vi "获取用户UID.vi"(8 "error in (no error)":errorcluster caption="错误输入（无错误）") -> (0 "error out":errorcluster caption="错误输出", 3 "uid":string[](array[string]))   [LabVIEW 2016, in "wxpusher.lvlib"]
uses:
  wxpusher.lvlib
  <vilib>/httpClient/LabVIEWHTTPClient.lvlib
panel:
  out "数据":T1
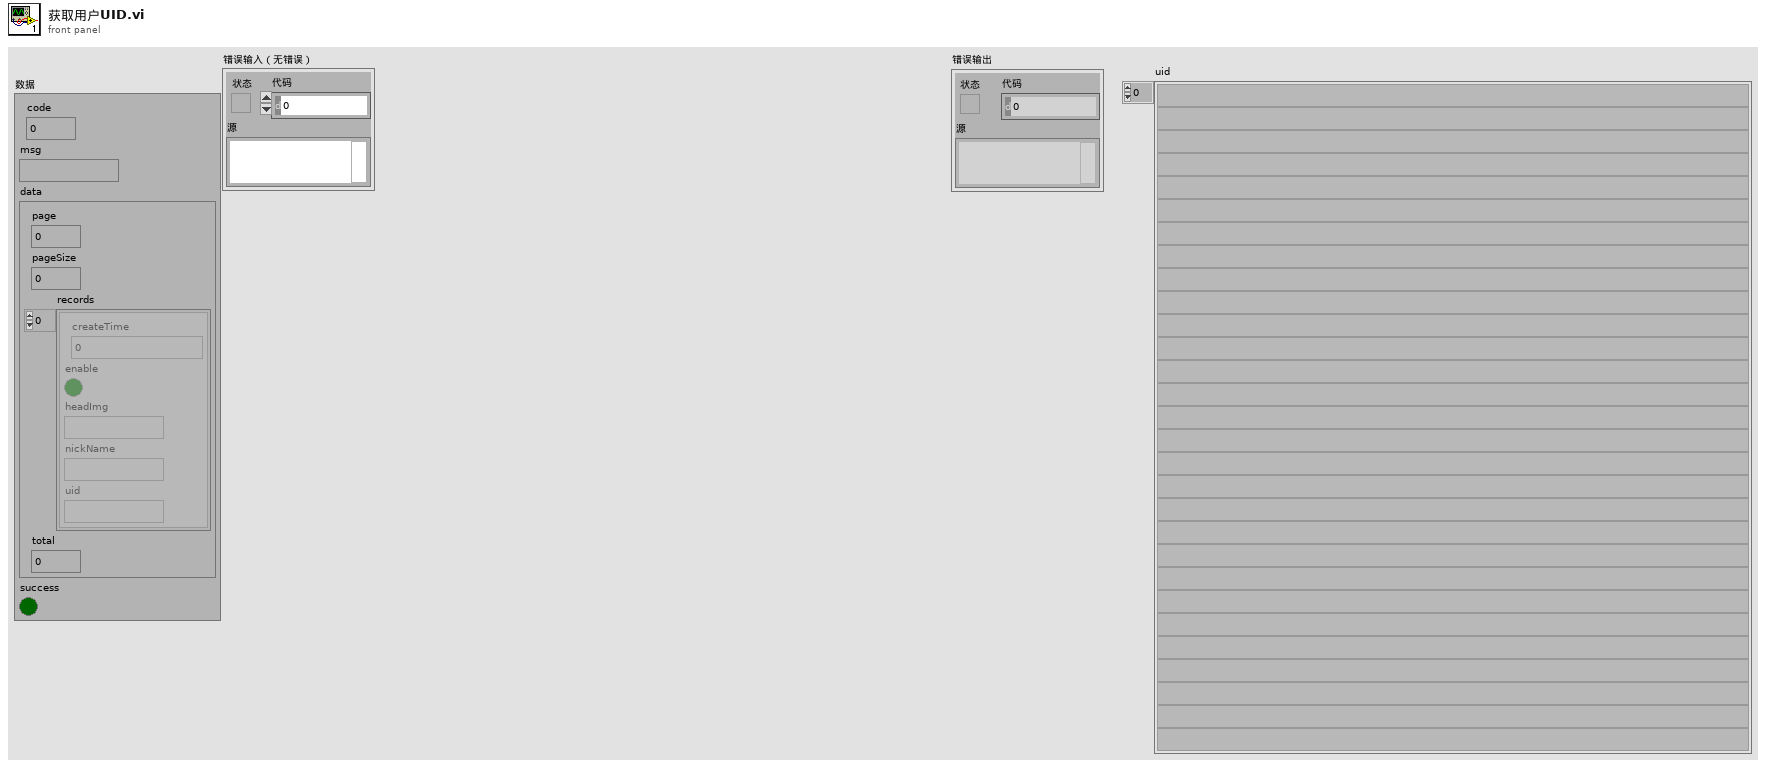
[diagram p1: front panel]
types:
  T1 = cluster{"code":i32, "msg":string, "data":cluster{"page":i32, "pageSize":i32, "records":cluster{"createTime":i32, "enable":bool, "headImg":string, "nickName":string, "uid":string}[], "total":i32}, "success":bool}
  T2 = cluster{"code":i32, "msg":string, "data":cluster{"page":i32, "pageSize":i32, "records":cluster{"createTime":u64, "enable":bool, "headImg":string, "nickName":string, "uid":string}[], "total":i32}, "success":bool}
  T3 = typedef "LabVIEWHTTPClient.lvlib/ClientHandle.ctl" = refnum<k1>
  T4 = cluster{"createTime":u64, "enable":bool, "headImg":string, "nickName":string, "uid":string}[]
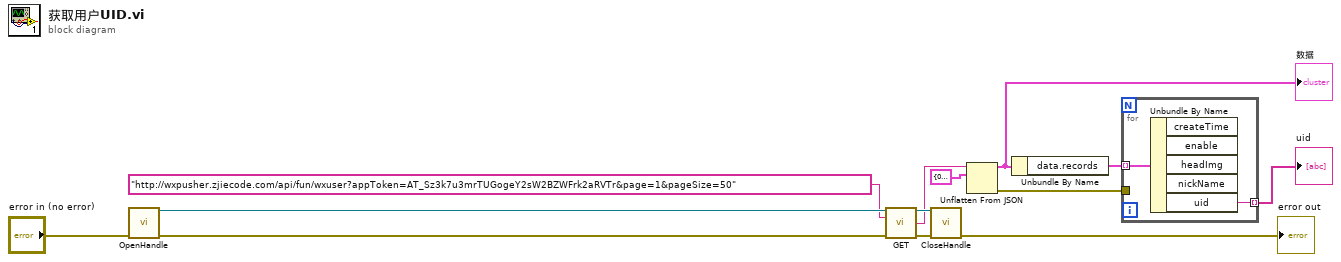
[diagram p0: block diagram]
diagram:
  n1 = call <vilib>:"OpenHandle.vi"("error in (no error)"="error in (no error)") -> ("client handle out"=w11:T3, "error out"=w10:errorcluster)  [unwired: 13 in]
  n2 = call <vilib>:"GET.vi"("client handle"=w11, "url"="http://wxpusher.zjiecode.com/api/fun/wxuser?appToken=AT_Sz3k7u3mrTUGogeY2sW2BZWFrk2aRVTr&page=1&pageSize=50", "error in (no error)"=w10) -> ("client handle out"=w12:T3, "body"=w7:string, "error out"=w13:errorcluster)  [unwired: 9 in, 1 out]
  n3 = call <vilib>:"CloseHandle.vi"("client handle"=w12, "error in (no error)"=w13) -> ("error out"=→"error out":errorcluster)  [unwired: 13 in]
  n4 = Unflatten From JSON(JSON string=w7, type and defaults=T2 {"code"=0, "msg"="", "data"={"page"=0, "pageSize"=0, "records"=[], "total"=0}, "success"=FALSE}) -> (value=w5:T2, error out=w1:errorcluster)  [unwired: 5 in]
  "数据" <- w5
  n5 = Unbundle By Name(w5) -> ("data.records"=w8:T4)
  n6 = for {
    tunnel: w8 -> [w15] mode=indexing
    tunnel: [w14] -> w4 mode=indexing
    tunnel: w1 -> [_]
    n7 = Unbundle By Name(w15) -> ("uid"=w14:string)  [unwired: 4 out]
  }
  "uid" <- w4
